vi "_Parse ACLR EN-DC Limit Check Result.vi"(8 "error in (no error)":errorcluster, 10 "Input String":string, 11 "VISA resource name":refnum<visa-resource-name>) -> (0 "error out":errorcluster, 1 "ACLR EN-DC Limit Check Results":T1, 2 "Reliability":i32, 3 "VISA resource name out":refnum<visa-resource-name>)   [LabVIEW 2020, in "Rohde&Schwarz CMWXP NR FR1 Measurement.lvlib"]
uses:
  <instrlib>/Rohde&Schwarz CMWXP NR FR1 Measurement/Rohde&Schwarz CMWXP NR FR1 Measurement.lvlib
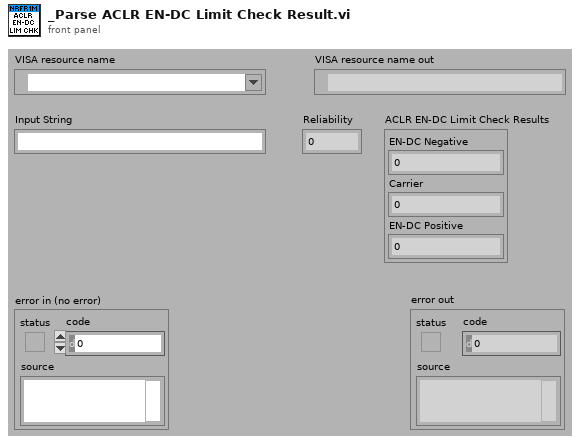
[diagram p1: front panel]
types:
  T1 = cluster{"EN-DC Negative":i32, "Carrier":i32, "EN-DC Positive":i32}
  T2 = cluster{"Limit Check Value":i32, "Limit Check Value":i32, "Limit Check Value":i32}
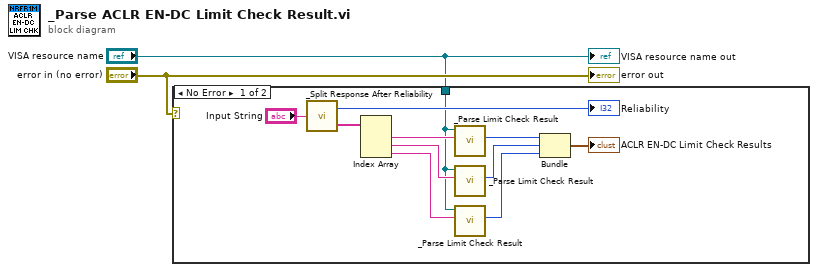
[diagram p0: block diagram]
diagram:
  n1 = case shown="No Error" "error in (no error)" {
    tunnel: "VISA resource name" -> [w4 _]
    frame No Error {
      n2 = call <instrlib>:"_Split Response After Reliability.vi"("Input String"="Input String") -> ("Response out"=w8:string[], "Reliability out"=→"Reliability":i32)
      n3 = Index Array(array=w8) -> (element #1=w7:string, element #2=w6:string, element #3=w5:string)  [unwired: 3 in]
      n4 = call <instrlib>:"_Parse Limit Check Result.vi"("String Value In"=w7, "VISA resource name"=w4) -> ("Limit Check Value"=w13:i32)  [unwired: 7 in, 2 out]
      n5 = call <instrlib>:"_Parse Limit Check Result.vi"("String Value In"=w6, "VISA resource name"=w4) -> ("Limit Check Value"=w12:i32)  [unwired: 7 in, 2 out]
      n6 = call <instrlib>:"_Parse Limit Check Result.vi"("String Value In"=w5, "VISA resource name"=w4) -> ("Limit Check Value"=w11:i32)  [unwired: 7 in, 2 out]
      n7 = Bundle("Limit Check Value"=w13, "Limit Check Value"=w12, "Limit Check Value"=w11) -> (→"ACLR EN-DC Limit Check Results":T2)  [unwired: 1 in]
    }
    frame Error {
    }
  }
  "VISA resource name out" <- "VISA resource name"
  "error out" <- "error in (no error)"
